vi "GetErrorControl.vi"(8 "error in (no error)":errorcluster, 10 "Name":string, 11 "VIEW in":refnum<class "VIEW.lvclass">) -> (0 "error out":errorcluster, 2 "error":errorcluster, 3 "VIEW out":refnum<class "VIEW.lvclass">)   [LabVIEW 2013, in "VIEW.lvclass"]
uses:
  VIEW.lvclass
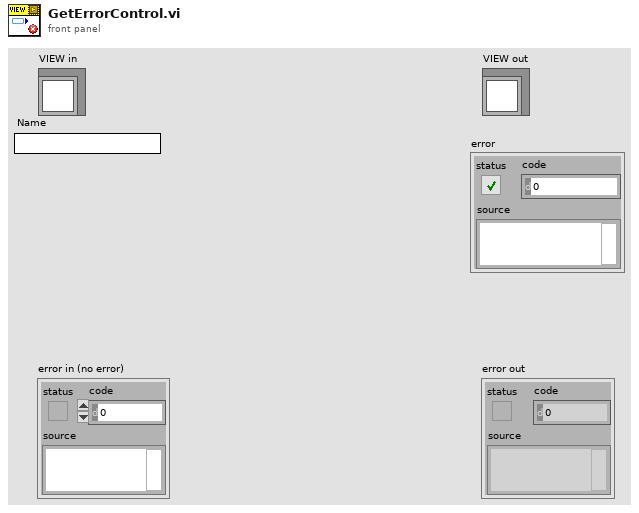
[diagram p1: front panel]
types:
  T1 = cluster{"CtlRef":refnum<vi>, "Name":string, "ClassName":string}
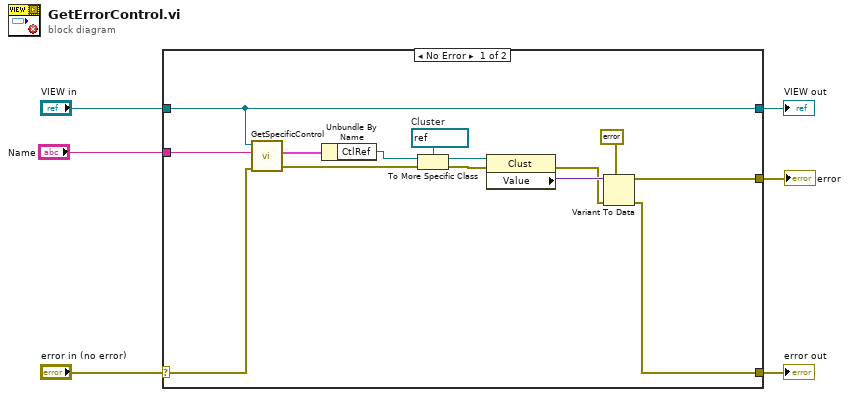
[diagram p0: block diagram]
diagram:
  n1 = case shown="No Error" "error in (no error)" {
    selector: "error in (no error)" -> [w15 w22]
    tunnel: [w8 w22] -> w5
    tunnel: [w20 w21] -> w3
    tunnel: "VIEW in" -> [w20 w21]
    tunnel: "Name" -> [w19 _]
    tunnel: [w7 _] -> w1
    frame No Error {
      w14 = refnum<vi> refnum  # Cluster
      n2 = call "GetSpecificControl.vi"("error in (no error)"=w15, "Name"=w19, "VIEW in"=w20) -> ("error out"=w16:errorcluster, "output cluster"=w17:T1)  [unwired: 6 in, 1 out]
      n3 = Unbundle By Name(w17) -> ("CtlRef"=w18:refnum<vi>)
      n4 = To More Specific Class(target class=w14, reference=w18, error in=w16) -> (specific class reference=w13:refnum<vi>, error out=w12:errorcluster)
      n5 = property class="Clust"(reference=w13, error in=w12) -> (error out=w9:errorcluster, "Value"=w11:variant)  [unwired: 1 out]
      n6 = Variant To Data(error in=w9, type=errorcluster {"status"=FALSE, "code"=0, "source"=""} ("error out"), Variant=w11) -> (data=w7:errorcluster, error out=w8:errorcluster)
    }
    frame Error {
    }
  }
  "error out" <- w5
  "VIEW out" <- w3
  "error" <- w1
